vi "commande_moteur.vi"(10 "liste commande":string[](array[string])) -> ()   [LabVIEW 2019]
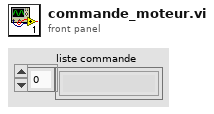
[diagram p1: front panel]
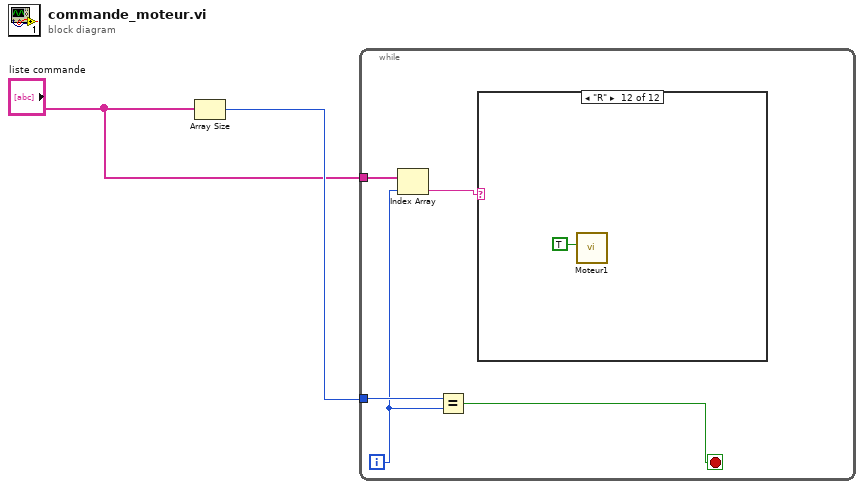
[diagram p0: block diagram]
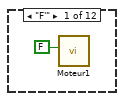
[diagram p2: hidden frame]
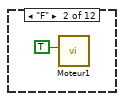
[diagram p3: hidden frame]
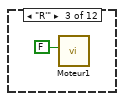
[diagram p4: hidden frame]
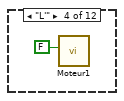
[diagram p5: hidden frame]
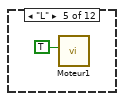
[diagram p6: hidden frame]
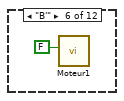
[diagram p7: hidden frame]
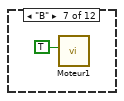
[diagram p8: hidden frame]
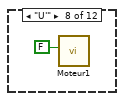
[diagram p9: hidden frame]
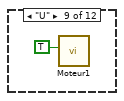
[diagram p10: hidden frame]
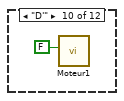
[diagram p11: hidden frame]
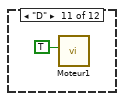
[diagram p12: hidden frame]
diagram:
  n1 = Array Size(array="liste commande") -> (size(s)=w2:i32)
  n2 = while {
    tunnel: w2 -> [w7]
    tunnel: "liste commande" -> [w4]
    i -> [w6]
    stop <- w5 stop-if-true
    n3 = Index Array(array=w4, index=w6) -> (element=w3:string)
    n4 = Equal?(x=w7, y=w6) -> (x = y?=w5:bool)
    n5 = case shown="\"R\"" w3 {
      frame "F'" {
        n6 = call "Moteur1.vi"("Sleep (A/DIO0 (Pin 11))"=FALSE ("DIR (A/DIO0 (Pin 11))")) -> ()  [unwired: 11 in]
      }
      frame "F" {
        n7 = call "Moteur1.vi"("Sleep (A/DIO0 (Pin 11))"=TRUE ("DIR (A/DIO0 (Pin 11))")) -> ()  [unwired: 11 in]
      }
      frame "R'" {
        n8 = call "Moteur1.vi"("Sleep (A/DIO0 (Pin 11))"=FALSE ("DIR (A/DIO0 (Pin 11))")) -> ()  [unwired: 11 in]
      }
      frame "L'" {
        n9 = call "Moteur1.vi"("Sleep (A/DIO0 (Pin 11))"=FALSE ("DIR (A/DIO0 (Pin 11))")) -> ()  [unwired: 11 in]
      }
      frame "L" {
        n10 = call "Moteur1.vi"("Sleep (A/DIO0 (Pin 11))"=TRUE ("DIR (A/DIO0 (Pin 11))")) -> ()  [unwired: 11 in]
      }
      frame "B'" {
        n11 = call "Moteur1.vi"("Sleep (A/DIO0 (Pin 11))"=FALSE ("DIR (A/DIO0 (Pin 11))")) -> ()  [unwired: 11 in]
      }
      frame "B" {
        n12 = call "Moteur1.vi"("Sleep (A/DIO0 (Pin 11))"=TRUE ("DIR (A/DIO0 (Pin 11))")) -> ()  [unwired: 11 in]
      }
      frame "U'" {
        n13 = call "Moteur1.vi"("Sleep (A/DIO0 (Pin 11))"=FALSE ("DIR (A/DIO0 (Pin 11))")) -> ()  [unwired: 11 in]
      }
      frame "U" {
        n14 = call "Moteur1.vi"("Sleep (A/DIO0 (Pin 11))"=TRUE ("DIR (A/DIO0 (Pin 11))")) -> ()  [unwired: 11 in]
      }
      frame "D'" {
        n15 = call "Moteur1.vi"("Sleep (A/DIO0 (Pin 11))"=FALSE ("DIR (A/DIO0 (Pin 11))")) -> ()  [unwired: 11 in]
      }
      frame "D" {
        n16 = call "Moteur1.vi"("Sleep (A/DIO0 (Pin 11))"=TRUE ("DIR (A/DIO0 (Pin 11))")) -> ()  [unwired: 11 in]
      }
      frame "R" {
        n17 = call "Moteur1.vi"("Sleep (A/DIO0 (Pin 11))"=TRUE ("DIR (A/DIO0 (Pin 11))")) -> ()  [unwired: 11 in]
      }
    }
  }
